vi "test Get Owning Disabled Custom Device.vi"(8 "error in":errorcluster, 11 "TestCase in":refnum<class "Scripting.lvclass">) -> (0 "error out":errorcluster, 3 "TestCase out":refnum<class "Scripting.lvclass">)   [LabVIEW 2020, in "Scripting.lvclass"]
uses:
  Scripting.lvclass
  Scripting.lvclass/Scripting.ctl
  Scripting/Ballard/Ballard ARINC 429 Scripting.lvlib
  <vilib>/addons/_JKI Toolkits/VI Tester/TestCase.llb/TestCase.lvclass
  C:/Program Files (x86)/National Instruments/LabVIEW 2020/vi.lib/addons/_JKI Toolkits/VI Tester/TestCase.llb/TestCase.lvclass
  C:/dev/git/niveristand-ballard-arinc429-custom-device/Source/Custom Device Support/Tests/Unit/Scripting/Scripting.lvclass
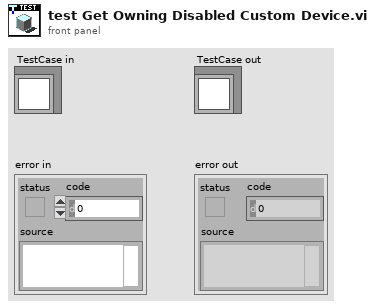
[diagram p1: front panel]
types:
  T1 = typedef "Custom Device API.lvlib/Custom Device Item Ref.ctl" = u64
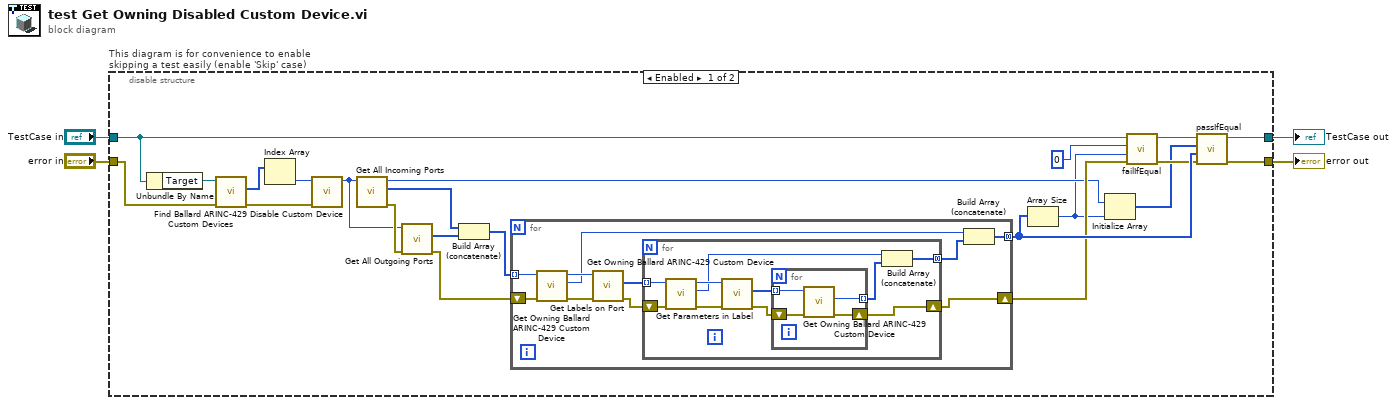
[diagram p0: block diagram]
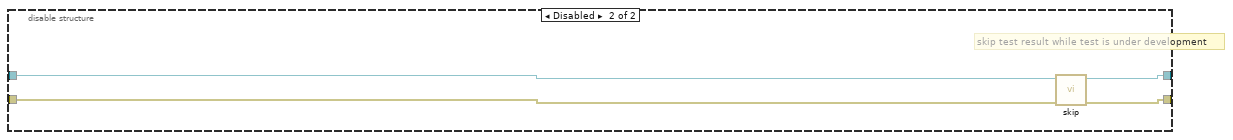
[diagram p2: hidden frame]
diagram:
  n1 = disable-structure "This diagram is for convenience to enable skipping a test easily (enable 'Skip' case)" shown="Enabled" {
    disable-tunnel: "TestCase in" -> [w6 w54]
    disable-tunnel: [w7 w52] -> w1
    disable-tunnel: [w25 w53] -> w3
    disable-tunnel: "error in" -> [w26 w51]
    frame Enabled {
      n2 = Unbundle By Name(w6) -> ("Target"=w13:refnum<k24>)
      n3 = call "Find Ballard ARINC-429 Custom Devices.vi"("error in"=w26, "target in"=w13) -> ("error out"=w14:errorcluster, "Ballard ARINC 429 custom devices"=w16:u64[])  [unwired: 7 in, 1 out]
      n4 = Index Array(array=w16) -> (element=w15:u64)  [unwired: 1 in]
      n5 = call "Disable Custom Device.vi"("error in (no error)"=w14, "Ballard ARINC 429 ref"=w15) -> ("Ballard ARINC 429 ref out"=w5:T1)  [unwired: 8 in, 1 out]
      n6 = call "Get All Incoming Ports.vi"("Ballard ARINC 429 custom device in"=w5) -> ("error out"=w12:errorcluster, "incoming ports"=w11:T1[], "Ballard ARINC 429 custom device out"=w19:T1)  [unwired: 8 in]
      n7 = call "Get All Outgoing Ports.vi"("error in"=w12, "Ballard ARINC 429 custom device in"=w5) -> ("error out"=w9:errorcluster, "outgoing ports"=w10:T1[])  [unwired: 7 in, 1 out]
      n8 = Build Array (concatenate)(w11, w10) -> (w8:T1[])
      n9 = for {
        tunnel: w8 -> [w36] mode=indexing
        shift-right: [w30] -> w21
        shift-left: w9 -> [w35]
        tunnel: [w27] -> w24 mode=concatenating
        n10 = call "Get Owning Ballard ARINC-429 Custom Device.vi"("error in"=w35, "item ref in"=w36) -> ("error out"=w33:errorcluster, "owning Ballard ARINC-429 custom device"=w28:T1, "item ref out"=w34:T1)  [unwired: 7 in]
        n11 = call "Get Labels on Port.vi"("error in"=w33, "port in"=w34) -> ("error out"=w31:errorcluster, "labels"=w32:T1[])  [unwired: 6 in, 2 out]
        n12 = for {
          tunnel: w32 -> [w46] mode=indexing
          shift-right: [w42] -> w30
          shift-left: w31 -> [w44]
          tunnel: [w37] -> w29 mode=concatenating
          n13 = call "Get Owning Ballard ARINC-429 Custom Device.vi"("error in"=w44, "item ref in"=w46) -> ("error out"=w43:errorcluster, "owning Ballard ARINC-429 custom device"=w39:T1, "item ref out"=w45:T1)  [unwired: 7 in]
          n14 = call "Get Parameters in Label.vi"("error in"=w43, "label in"=w45) -> ("error out"=w40:errorcluster, "parameters"=w41:T1[])  [unwired: 6 in, 2 out]
          n15 = for {
            tunnel: w41 -> [w50] mode=indexing
            tunnel: [w49] -> w38 mode=indexing
            shift-right: [w47] -> w42
            shift-left: w40 -> [w48]
            n16 = call "Get Owning Ballard ARINC-429 Custom Device.vi"("error in"=w48, "item ref in"=w50) -> ("error out"=w47:errorcluster, "owning Ballard ARINC-429 custom device"=w49:T1)  [unwired: 7 in, 1 out]
          }
          n17 = Build Array (concatenate)(w39, w38) -> (w37:T1[])
        }
        n18 = Build Array (concatenate)(w28, w29) -> (w27:T1[])
      }
      n19 = Array Size(array=w24) -> (size(s)=w18:i32)
      n20 = Initialize Array(w19, w18) -> (w17:T1[])
      n21 = call-dynamic "failIfEqual.vi"("error in (no error)"=w21, "y"=w18, "x"=0 ("size(s)"), "TestCase in"=w6) -> ("error out"=w20:errorcluster, "TestCase out"=w22:refnum<class "Scripting.lvclass">)  [unwired: 6 in]
      n22 = call-dynamic "passIfEqual.vi"("error in (no error)"=w20, "y"=w24, "x"=w17, "TestCase in"=w22) -> ("error out"=w25:errorcluster, "TestCase out"=w7:refnum<class "Scripting.lvclass">)  [unwired: 6 in]
    }
    frame Disabled {
      # "skip test result while test is under development"
      n23 = call <vilib>:"skip.vi"("error in (no error)"=w51, "TestCase in"=w54) -> ("error out"=w53:errorcluster, "TestCase out"=w52:refnum<class "Scripting.lvclass">)  [unwired: 8 in]
    }
  }
  "error out" <- w3
  "TestCase out" <- w1
